vi "q(i).vi"(0 "Amplitude":dbl, 1 "N":dbl[](array[numeric]), 5 "beta":dbl, 7 "sigma":dbl, 9 "T(0) [dB]":dbl, 11 "Response":bool, 12 "offset":dbl format="%#_13g") -> (4 "q(i)":cluster{"Ramp Pattern":dbl[], "Y":dbl[]}(graph), 6 "likehood function":cluster{"Ramp Pattern":dbl[], "y":dbl[]}(graph), 10 "T(i)":dbl, 15 "q(i)":dbl[](array[numeric]))   [LabVIEW 2022 SP3]
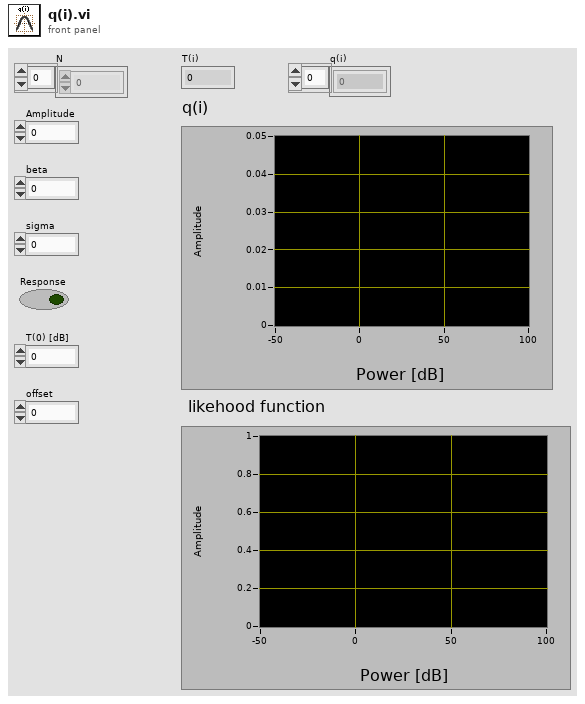
[diagram p1: front panel]
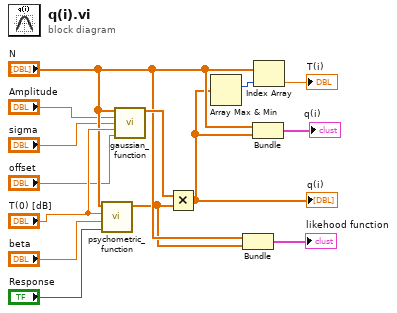
[diagram p0: block diagram]
diagram:
  n1 = call "psychometric_function.vi"("Response"="Response", "beta"="beta", "T(i)"="T(0) [dB]", "N"="N") -> ("S(response, N)"=w4:dbl[])  [unwired: 6 in]
  n2 = call "gaussian_function.vi"("X"="N", "Amplitude"="Amplitude", "sigma"="sigma", "mean"="T(0) [dB]", "offset"="offset") -> ("Y"=w10:dbl[])  [unwired: 10 in]
  n3 = Multiply(x=w10, y=w4) -> (x*y=w6:dbl[])
  "q(i)" <- w6
  n4 = Array Max & Min(array=w6) -> (max index (indices)=w3:i32)  [unwired: 3 out]
  n5 = Bundle("N"="N", "S(response, N)"=w4) -> (→"likehood function":cluster{"N":dbl[], "S(response, N)":dbl[]})  [unwired: 1 in]
  n6 = Bundle("N"="N", w6) -> (→"q(i)":cluster{"N":dbl[], dbl[]})  [unwired: 1 in]
  n7 = Index Array(array="N", index=w3) -> (element=→"T(i)":dbl)
